vi "FL_Last_N_Samples_1D.vi"(1 "BufferLengthSamples":u32=100, 2 "Input Array":dbl[](array[numeric])) -> (0 "Output Array":dbl[](array[numeric]))   [LabVIEW 2018, in "Tracker.lvlib"]
uses:
  Tracker.lvlib
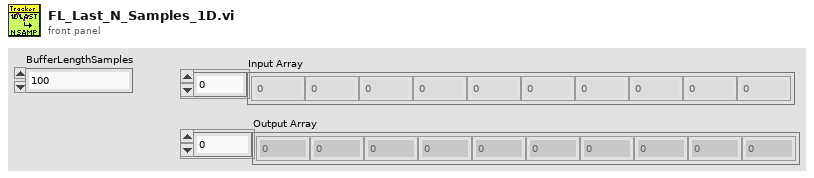
[diagram p1: front panel]
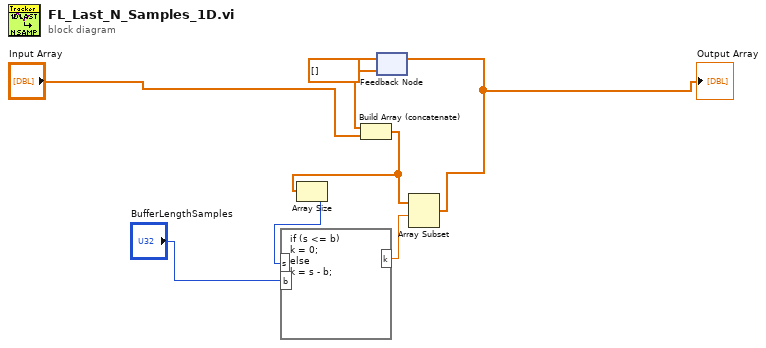
[diagram p0: block diagram]
diagram:
  n1 = feedback #1(dbl[] []) -> (w8:dbl[])
  n2 = Build Array (concatenate)(w8, "Input Array") -> (w7:dbl[])
  n3 = Array Size(array=w7) -> (size(s)=w6:i32)
  n4 = formula code="if (s <= b)\nk = 0;\nelse\nk = s - b;"("s"=w6, "b"="BufferLengthSamples") -> ("k"=w5:dbl)
  n5 = Array Subset(array=w7, index=w5) -> (w2:dbl[])  [unwired: 1 in]
  "Output Array" <- w2
  n6 = feedback-in #1(w2) -> ()
